vi "Residue.vi"(6 "residue":dbl, 8 "Current Interval":i32, 10 "Linear Fit \nResidue Threshold":dbl=2.0 format="%.3g", 11 "None linear \nIntervals IN":dbl[](array[numeric])) -> (3 "None linear \nIntervals OUT":dbl[](array[numeric]))   [LabVIEW 2014]
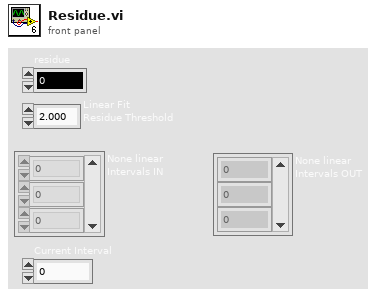
[diagram p1: front panel]
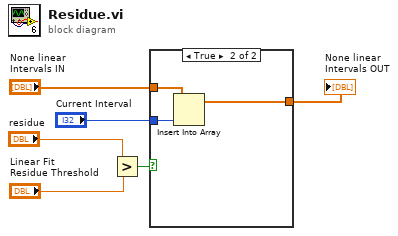
[diagram p0: block diagram]
diagram:
  n1 = Greater?(x="residue", y="Linear Fit \nResidue Threshold") -> (0:w3:bool)
  n2 = case shown="True" w3 {
    tunnel: "None linear \nIntervals IN" -> [w7 w10]
    tunnel: "Current Interval" -> [_ w9]
    tunnel: [w7 w8] -> w1
    frame False {
    }
    frame True {
      n3 = Insert Into Array(array=w10, new element=w9) -> (w8:dbl[])  [unwired: 1 in]
    }
  }
  "None linear \nIntervals OUT" <- w1
